vi "Step Core.vi"(8 "error in (no error)":errorcluster, 11 "QPA Measurement in":refnum<class "QPA Measurement.lvclass">) -> (0 "error out":errorcluster, 2 "Step Out":refnum<k7>, 3 "QPA Measurement out":refnum<class "QPA Measurement.lvclass">)   [LabVIEW 2016, in "QPA Measurement.lvlib" / "QPA Measurement.lvclass"]
uses:
  QPA Measurement.lvclass
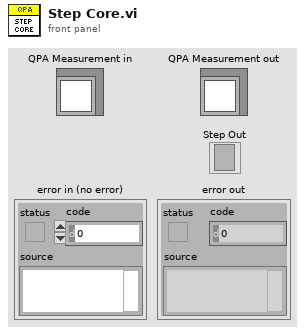
[diagram p1: front panel]
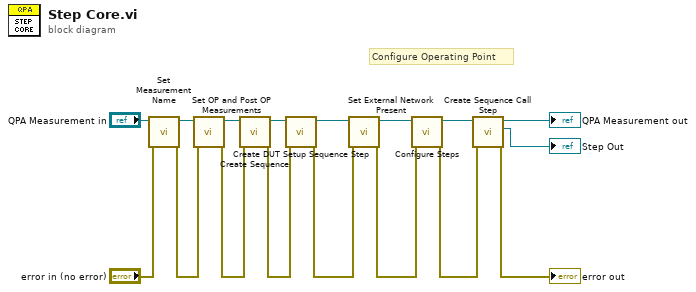
[diagram p0: block diagram]
diagram:
  # "Configure Operating Point"
  n1 = call-dynamic "Set Measurement Name.vi"("error in (no error)"="error in (no error)", "QPA Measurement in"="QPA Measurement in") -> ("error out"=w16:errorcluster, "QPA Measurement out"=w5:refnum<class "QPA Measurement.lvclass">)  [unwired: 8 in]
  n2 = call-dynamic "Set OP and Post OP Measurements.vi"("error in (no error)"=w16, "QPA Measurement in"=w5) -> ("error out"=w6:errorcluster, "QPA Measurement out"=w4:refnum<class "QPA Measurement.lvclass">)  [unwired: 8 in]
  n3 = call "Create Sequence.vi"("error in (no error)"=w6, "QPA Measurement in"=w4) -> ("error out"=w14:errorcluster, "QPA Measurement out"=w7:refnum<class "QPA Measurement.lvclass">)  [unwired: 8 in]
  n4 = call "Create DUT Setup Sequence Step.vi"("error in (no error)"=w14, "QPA Measurement in"=w7) -> ("error out"=w8:errorcluster, "QPA Measurement out"=w2:refnum<class "QPA Measurement.lvclass">)  [unwired: 8 in]
  n5 = call "Set External Network Present.vi"("error in (no error)"=w8, "QPA Measurement in"=w2) -> ("error out"=w3:errorcluster, "QPA Measurement out"=w1:refnum<class "QPA Measurement.lvclass">)  [unwired: 8 in]
  n6 = call-dynamic "Configure Steps.vi"("error in (no error)"=w3, "QPA Measurement in"=w1) -> ("error out"=w10:errorcluster, "QPA Measurement out"=w9:refnum<class "QPA Measurement.lvclass">)  [unwired: 8 in]
  n7 = call "Create Sequence Call Step.vi"("error in (no error)"=w10, "QPA Measurement in"=w9) -> ("error out"=→"error out":errorcluster, "Step Reference"=→"Step Out":refnum<k7>, "QPA Measurement out"=→"QPA Measurement out":refnum<class "QPA Measurement.lvclass">)  [unwired: 7 in]
